vi "Get Azimut and FOV.vi"(4 "Transformation Matrix":T1, 6 "Image Size [pix]":cluster{"Width":u32, "Height":u32}, 7 "Axial Distance [um]":dbl, 8 "Final Reference Point [um]":cluster{"X":dbl, "Y":dbl}, 9 "Initial Reference Point [um]":cluster{"X":dbl, "Y":dbl}, 10 "Final Visual Point[pix]":cluster{"X":sgl, "Y":sgl}, 11 "Initial Visual Point [pix]":cluster{"X":sgl, "Y":sgl}) -> (1 "Angle [deg]":dbl, 2 "Angle [rad]":dbl, 3 "FOV [um]":cluster{"Width":dbl, "Height":dbl})   [LabVIEW 2012, in "Targeting Unit.lvlib"]
uses:
  Targeting Unit.lvlib
  <vilib>/Analysis/Matrix/Datatypes/RealMatrix.ctl
  <vilib>/Analysis/Matrix/NI_Matrix.lvlib
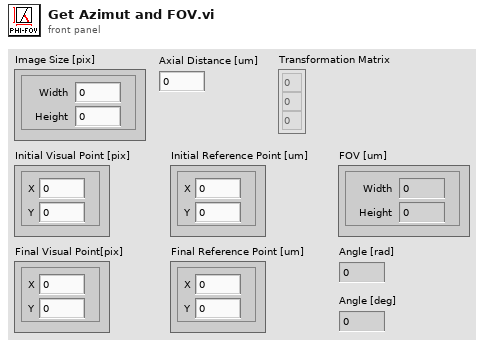
[diagram p1: front panel]
types:
  T1 = typedef "NI_Matrix.lvlib/RealMatrix.ctl" = dbl[][]
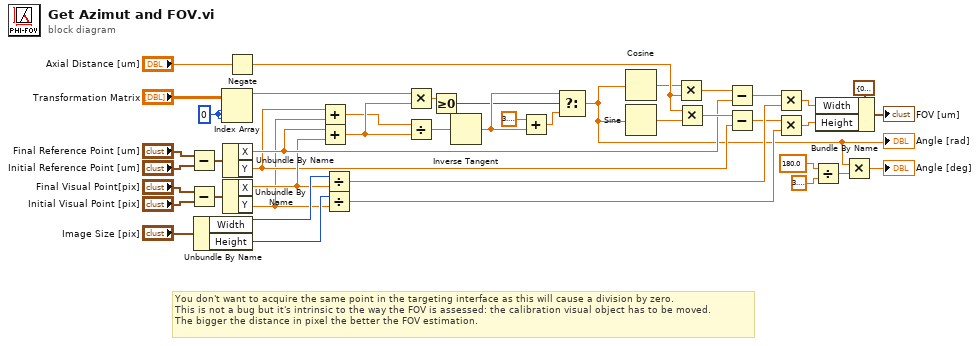
[diagram p0: block diagram]
diagram:
  w41 = 0 ("index (row)")
  # "You don't want to acquire the same point in the targeting interface as this will cause a division by zero.\nThis is not a bug but it's intrinsic to the way the FOV is assessed: the calibration visual object has to be moved.\nThe bigger the distance in pixel the better the FOV estimation."
  n1 = Subtract(x="Final Reference Point [um]", y="Initial Reference Point [um]") -> (x-y=w18:cluster{"X":dbl, "Y":dbl})
  n2 = Subtract(x="Final Visual Point[pix]", y="Initial Visual Point [pix]") -> (x-y=w31:cluster{"X":sgl, "Y":sgl})
  n3 = Unbundle By Name("Image Size [pix]") -> ("Width"=w34:u32, "Height"=w35:u32)
  n4 = Index Array(array="Transformation Matrix", index (row)=w41, index (col)=w41) -> (element=w43:dbl)
  n5 = Unbundle By Name(w18) -> ("X"=w11:dbl, "Y"=w9:dbl)
  n6 = Unbundle By Name(w31) -> ("X"=w10:sgl, "Y"=w8:sgl)
  n7 = Negate(x="Axial Distance [um]") -> (-x=w28:dbl)
  n8 = Add(x=w9, y=w8) -> (x+y=w6:dbl)
  n9 = Add(x=w11, y=w10) -> (x+y=w7:dbl)
  n10 = Divide(x=w34, y=w10) -> (x/y=w15:sgl)
  n11 = Divide(x=w35, y=w8) -> (x/y=w14:sgl)
  n12 = Multiply(x=w43, y=w7) -> (x*y=w40:dbl)
  n13 = Divide(x=w6, y=w7) -> (x/y=w27:dbl)
  n14 = Greater Or Equal To 0?(x=w40) -> (x >= 0?=w24:bool)
  n15 = Inverse Tangent(1:w27) -> (0:w25:dbl)
  n16 = Add(x=3.141592653589793, y=w25) -> (x+y=w23:dbl)
  n17 = Select(t=w25, s=w24, f=w23) -> (s? t:f=w2:dbl)
  "Angle [rad]" <- w2
  n18 = Cosine(x=w2) -> (cos(x)=w22:dbl)
  n19 = Sine(x=w2) -> (sin(x)=w21:dbl)
  n20 = Multiply(x=w22, y=w28) -> (x*y=w17:dbl)
  n21 = Multiply(x=w28, y=w21) -> (x*y=w16:dbl)
  n22 = Subtract(x=w17, y=w11) -> (x-y=w13:dbl)
  n23 = Subtract(x=w16, y=w9) -> (x-y=w12:dbl)
  n24 = Multiply(x=w13, y=w15) -> (x*y=w39:dbl)
  n25 = Multiply(x=w12, y=w14) -> (x*y=w38:dbl)
  n26 = Divide(x=180.0, y=3.141592653589793) -> (x/y=w3:dbl)
  n27 = Bundle By Name(cluster=cluster{"Width":dbl, "Height":dbl} {"Width"=0.0, "Height"=0.0} ("FOV [um]"), "Width"=w39, "Height"=w38) -> (→"FOV [um]":cluster{"Width":dbl, "Height":dbl})
  n28 = Multiply(x=w2, y=w3) -> (x*y=→"Angle [deg]":dbl)
